vi "VALEW_ATC_Calc Valve on times.vi"(0 "V(segment)":dbl, 5 "T(segment target)":dbl, 9 "T(cold inlet)":dbl, 11 "T(hot inlet)":dbl) -> (6 "t(hot valve)":u16, 10 "t(cold valve)":u16)   [LabVIEW 2016, in "TL27.lvlib"]
uses:
  Projects/TL27.lvlib
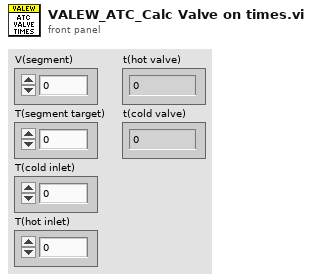
[diagram p1: front panel]
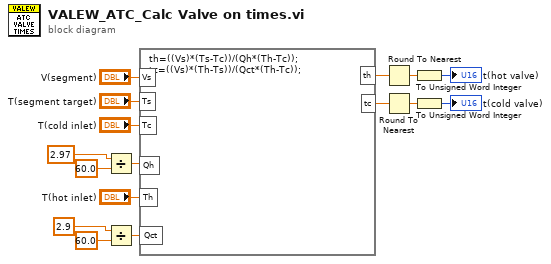
[diagram p0: block diagram]
diagram:
  n1 = Divide(x=2.97 ("input variable"), y=60.0) -> (x/y=w7:dbl)
  n2 = Divide(x=2.9 ("input variable"), y=60.0) -> (x/y=w9:dbl)
  n3 = formula code="th=((Vs)*(Ts-Tc))/(Qh*(Th-Tc));\ntc=((Vs)*(Th-Ts))/(Qct*(Th-Tc));"("Vs"="V(segment)", "Ts"="T(segment target)", "Tc"="T(cold inlet)", "Qh"=w7, "Th"="T(hot inlet)", "Qct"=w9) -> ("th"=w6:dbl, "tc"=w5:dbl)
  n4 = Round To Nearest(number=w6) -> (nearest integer value=w3:dbl)
  n5 = Round To Nearest(number=w5) -> (nearest integer value=w2:dbl)
  n6 = To Unsigned Word Integer(number=w3) -> (unsigned 16bit integer=→"t(hot valve)":u16)
  n7 = To Unsigned Word Integer(number=w2) -> (unsigned 16bit integer=→"t(cold valve)":u16)
